vi "FTW-Ether-Instance.vi"() -> ()   [LabVIEW 2013, in "FTW-Ether.lvclass"]
uses:
  FTW-Ether.lvclass
  EventLogger/FTW-Logger.lvclass
panel:
  in  "Application Version":string
  in  "Application Name":string
  in  "Logger Address":string
  in  "Default Linger":i32=500 format="%dmsec"
  in  "ØMQ Context":u64 format="%016x"
  in  "Logger":refnum<class "FTW-Logger.lvclass">
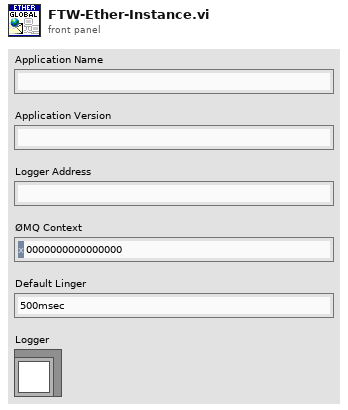
[diagram p1: front panel]
diagram:
